vi "Show Read Only Console.vi"(11 "Show Console":bool) -> (3 "VI out":refnum<vi>)   [LabVIEW 2017, in "Communications Console Library.lvlib"]
uses:
  Console GUI (Read-Only).vi
  Communications Console Library.lvlib
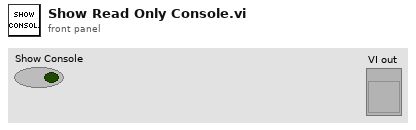
[diagram p1: front panel]
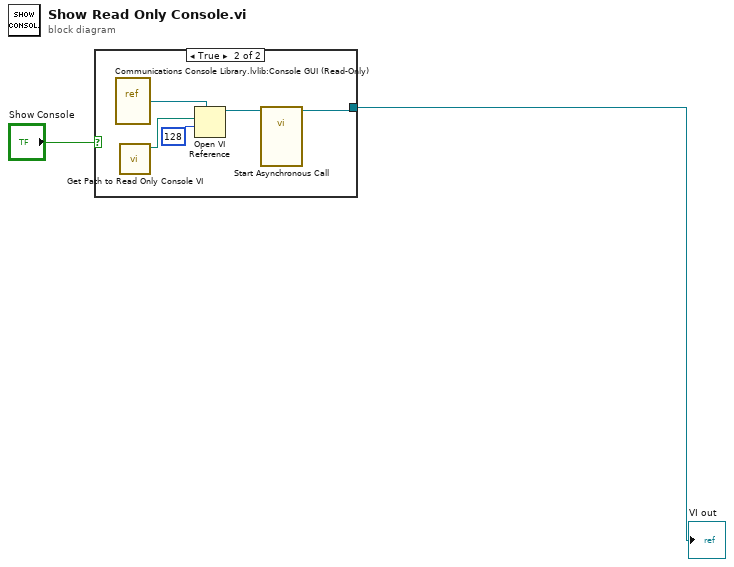
[diagram p0: block diagram]
diagram:
  n1 = case shown="True" "Show Console" {
    tunnel: [_ w4] -> w2
    frame False {
    }
    frame True {
      n2 = vi-ref "Communications Console Library.lvlib:Console GUI (Read-Only).vi"() -> (w7:refnum<vi>)
      n3 = call "Get Path to Read Only Console VI.vi"() -> ("Console VI Path"=w6:path)  [unwired: 11 in]
      n4 = Open VI Reference(type specifier VI Refnum (for type only)=w7, vi path=w6, options=128) -> (vi reference=w5:refnum<vi>)  [unwired: 3 in, 1 out]
      n5 = call-by-ref "Start Asynchronous Call"(reference=w5) -> (reference out=w4:refnum<vi>)  [unwired: 13 in, 1 out]
    }
  }
  "VI out" <- w2
